vi "SetDcOffset.vi"(8 "error in (no error)":errorcluster, 9 "FPGA Setting":T1=enum."DC_offs 1", 10 "DC offset":dbl caption="DC offset\nChannel 1", 11 "FpgaRef5761 In":refnum<class "FpgaRef5761.lvclass">) -> (0 "error out":errorcluster, 3 "FpgaRef5761 Out":refnum<class "FpgaRef5761.lvclass">)   [LabVIEW 2018, in "FpgaRef5761.lvclass"]
uses:
  FpgaRef5761.lvclass
  FPGA/fpga_settings.ctl
  <vilib>/rvi/FXPMathLib/FxpInterpret/XNode/nifxpmath_Interpret.xnode
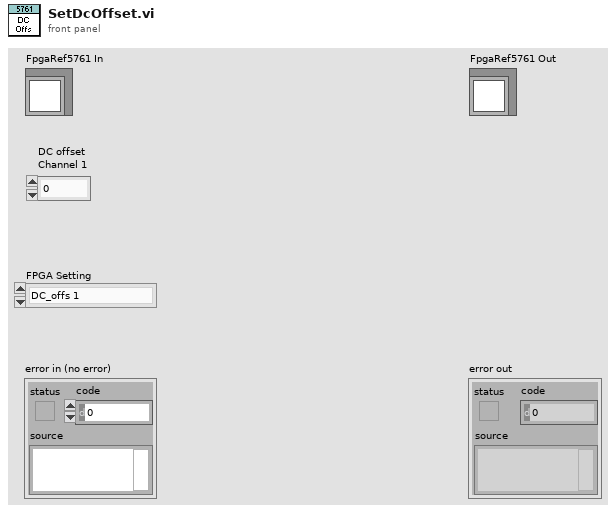
[diagram p1: front panel]
types:
  T1 = typedef "fpga_settings.ctl" = enum16{"Feedback Enable", "New FIR coeffs", "FIR shift", "Enable filter", "Set Downsample", "Downsample", "CIC Gain", "Record length", "Trigger samples", "Quiet time", "a_am", "b_am", "Use fixed delay", "fixed sin_fi", "fixed cos_fi", "Ki*Tau", "Kp", "Kd_Tau", "Fi_start", "Fi_delta", "DC_offs 0", "DC_offs 1", "DC_offs 2", "DC_offs 3", "Ki*Tau am", "Kp am", "Kd_Tau am", "Feedback AM", "Trigger delay", "Feedback delay", "Setpoint enable", "Beam enable", "Samples to acquire", "Cavity Enable", "Cavity C1", "Cavity C2", "Cavity C3", "Cavity C4", "Cavity C5"}
  T2 = typedef "settingsFPGAref.ctl" = refnum<k20>
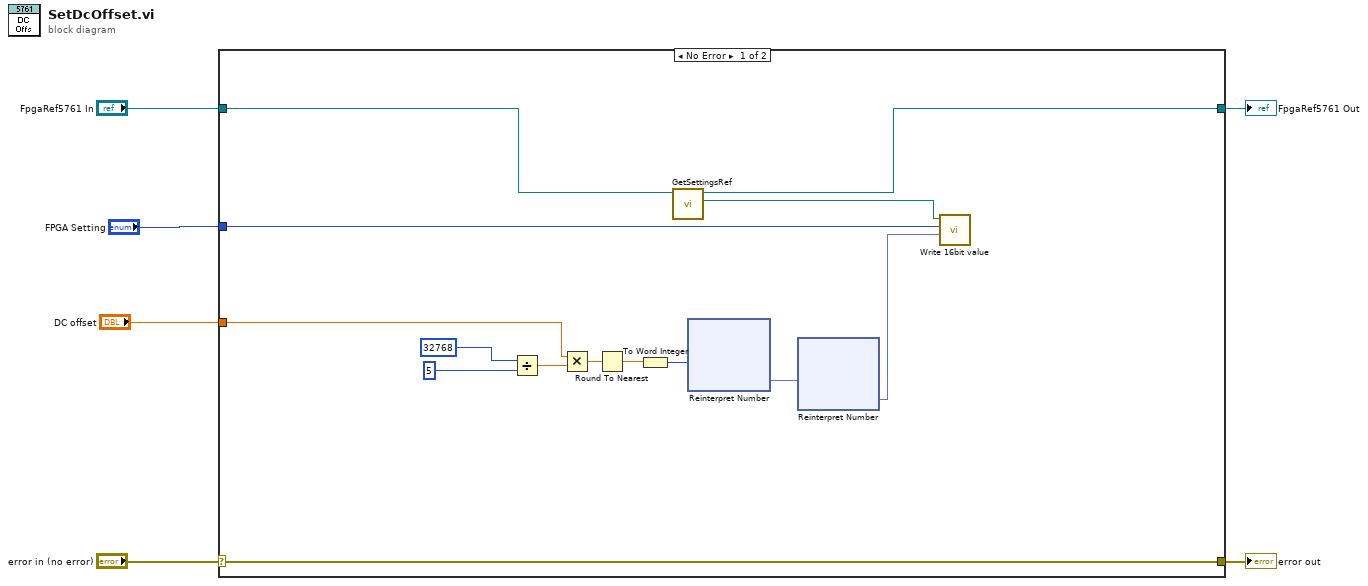
[diagram p0: block diagram]
diagram:
  n1 = case shown="No Error" "error in (no error)" {
    selector: "error in (no error)" -> [w20 w22]
    tunnel: [w20 w22] -> w5
    tunnel: [w10 w21] -> w3
    tunnel: "FpgaRef5761 In" -> [w9 w21]
    tunnel: "DC offset" -> [w8 _]
    tunnel: "FPGA Setting" -> [w7 _]
    frame No Error {
      n2 = Divide(x=32768, y=5) -> (x/y=w18:dbl)
      n3 = Multiply(x=w8, y=w18) -> (x*y=w17:dbl)
      n4 = Round To Nearest(number=w17) -> (nearest integer value=w16:dbl)
      n5 = To Word Integer(number=w16) -> (16bit integer=w12:i16)
      n6 = call-dynamic "GetSettingsRef.vi"("FpgaRef5761 in"=w9) -> ("Settings FPGA ref"=w11:T2, "FpgaRef5761 out"=w10:refnum<class "FpgaRef5761.lvclass">)  [unwired: 8 in, 1 out]
      n7 = xnode "Reinterpret Number"("x"=w12) -> ("y"=w14:fxp<+/-,16,14>)
      n8 = xnode "Reinterpret Number"("x"=w14) -> ("y"=w13:fxp<+,16,16>)
      n9 = call "Write 16bit value.vi"("value"=w13, "FPGA Setting"=w7, "FPGA ref"=w11) -> ()  [unwired: 7 in, 2 out]
    }
    frame Error {
    }
  }
  "error out" <- w5
  "FpgaRef5761 Out" <- w3
